vi "CTRE_PigeonIMU_RefNumRegistryGet.vi"(8 "error in (no error)":errorcluster, 10 "refnum name":string="My Pigeon RefNum") -> (0 "error out":errorcluster, 3 "PigeonIMUDevRef":T1={"DeviceStatus"={"status"=FALSE, "code"=0, "source"=""}, "Device Number"=0, "Type"=352321536, "Device ID"=0, "Handle"=0, "UsageFrame"=0, "Library Path"=path ""} {"Type" items=["CAN"=352321536, "TalonSRX"=33554432]})   [LabVIEW 2017]
uses:
  CTRE_PigeonIMU_DeviceRef.ctl
  CTRE_PigeonIMU_ConnectionType.ctl
  <vilib>/Rock Robotics/WPI/Utilities/Refnum Registry Operation.ctl
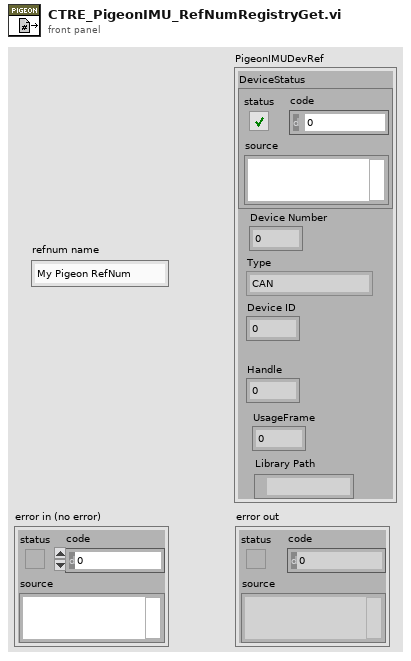
[diagram p1: front panel]
types:
  T1 = typedef "CTRE_PigeonIMU_DeviceRef.ctl" = cluster{"DeviceStatus":errorcluster, "Device Number":u8, "Type":T2, "Device ID":u32, "Handle":u64, "UsageFrame":u32, "Library Path":path}
  T2 = typedef "CTRE_PigeonIMU_ConnectionType.ctl" = u32
  T3 = typedef "Refnum Registry Operation.ctl" = enum16{"set", "get", "delete", "get all names", "read name"}
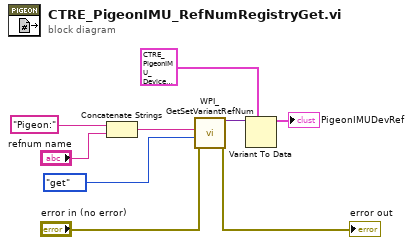
[diagram p0: block diagram]
diagram:
  n1 = Concatenate Strings("Pigeon:", "refnum name") -> (w9:string)
  n2 = call <vilib>:"WPI_GetSetVariantRefNum.vi"("error in (no error)"="error in (no error)", "Operation"=Refnum_Registry_Operation."get" ("menu"), "refnum name"=w9) -> ("error out"=→"error out":errorcluster, "DevRef"=w8:variant)  [unwired: 6 in, 1 out]
  n3 = Variant To Data(type=T1 {"DeviceStatus"={"status"=FALSE, "code"=0, "source"=""}, "Device Number"=0, "Type"=352321536, "Device ID"=0, "Handle"=0, "UsageFrame"=0, "Library Path"=path ""} ("PigeonIMUDevRef"), Variant=w8) -> (data=→"PigeonIMUDevRef":T1)  [unwired: 1 in, 1 out]
